vi "Vision Targeting.vi"(6 "reinitialize?":bool, 10 "output range":cluster{"output high":dbl, "output low":dbl}={"output high"=1.0, "output low"=-1.0} {"output low" format="%.2f"; "output high" format="%.2f"}, 11 "PID gains":T1={"proportional gain (Kc)"=0.1, "integral time (Ti, min)"=0.0, "derivative time (Td, min)"=0.0} {"derivative time (Td, min)" format="%.3f"; "integral time (Ti, min)" format="%.3f"; "proportional gain (Kc)" format="%.3f"}) -> (1 "Azimuth Ready":bool, 3 "X Axis output":dbl)   [LabVIEW 2013]
uses:
  Robot Global Data.vi
  <vilib>/addons/control/pid/pid.llb/PID (DBL).vi
  <vilib>/addons/control/pid/NI_PID_pid.lvlib
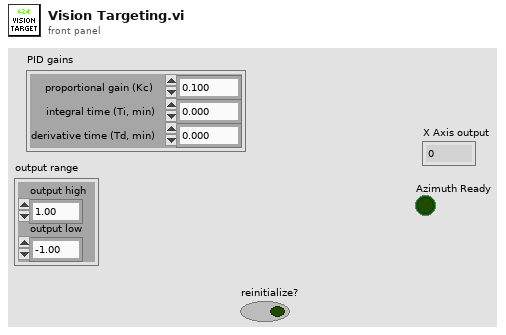
[diagram p1: front panel]
types:
  T1 = cluster{"proportional gain (Kc)":dbl, "integral time (Ti, min)":dbl, "derivative time (Td, min)":dbl}
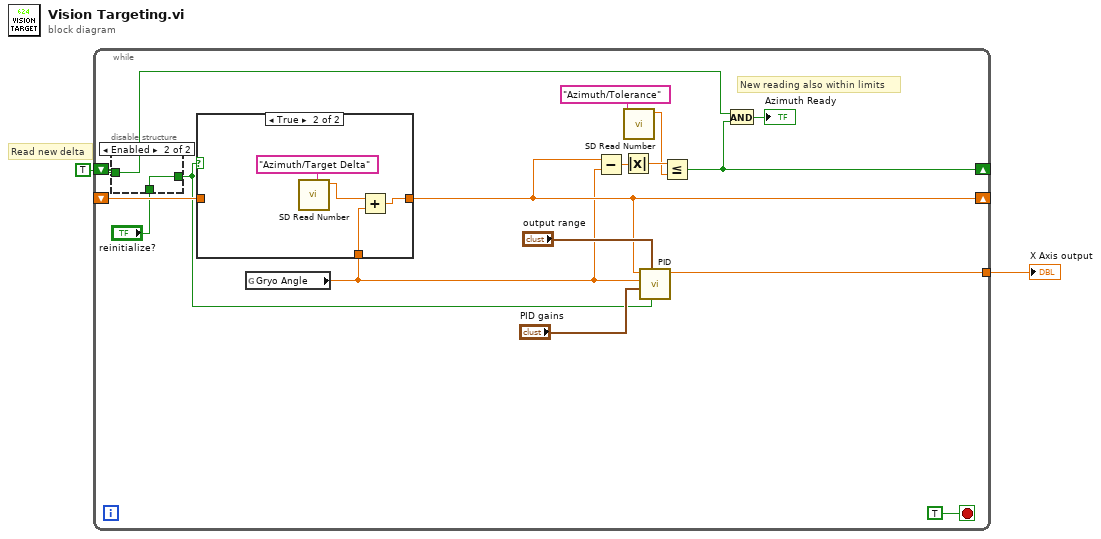
[diagram p0: block diagram]
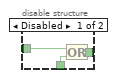
[diagram p2: hidden frame]
diagram:
  # "Read new delta"
  n1 = while {
    shift-right: [w3] -> _
    shift-left: TRUE -> [w4]
    shift-right: [w12] -> _
    shift-left: _ -> [w17]
    tunnel: [w16] -> w1
    stop <- TRUE stop-if-true
    # "New reading also within limits"
    n2 = disable-structure shown="Enabled" {
      disable-tunnel: [w21 w22] -> w7
      disable-tunnel: "reinitialize?" -> [w20 w22]
      disable-tunnel: w4 -> [w19 _]
      frame Disabled {
        n3 = Or(x=w19, y=w20) -> (x .or. y?=w21:bool)
      }
      frame Enabled {
      }
    }
    n4 = global read "Robot Global Data.vi" "Gryo Angle"() -> (w8:dbl)
    n5 = case shown="True" w7 {
      tunnel: [w23 w24] -> w12
      tunnel: w17 -> [w23 _]
      tunnel: w8 -> [_ w26]
      frame False {
      }
      frame True {
        n6 = call <vilib>:"SD Read Number.vi"("Name"="Azimuth/Target Delta") -> ("Numeric"=w25:dbl)  [unwired: 8 in, 2 out]
        n7 = Add(x=w25, y=w26) -> (x+y=w24:dbl)
      }
    }
    n8 = Subtract(x=w12, y=w8) -> (x-y=w13:dbl)
    n9 = Absolute Value(x=w13) -> (abs(x)=w11:dbl)
    n10 = call <vilib>:"SD Read Number.vi"("Name"="Azimuth/Tolerance") -> ("Numeric"=w9:dbl)  [unwired: 8 in, 2 out]
    n11 = call-poly <vilib>:"PID.vi"("reinitialize? (F)"=w7, "output range"="output range", "PID gains"="PID gains", "process variable"=w8, "setpoint"=w12) -> ("output"=w16:dbl)  [unwired: 5 in, 1 out]
    n12 = Less Or Equal?(x=w11, y=w9) -> (x <= y?=w3:bool)
    n13 = And(x=w4, y=w3) -> (x .and. y?=→"Azimuth Ready":bool)
  }
  "X Axis output" <- w1
